vi "Clenshaw.vi"(10 "Cheby weights":dbl[](array[numeric]), 11 "x":dbl) -> (3 "y":dbl)   [LabVIEW 2019]
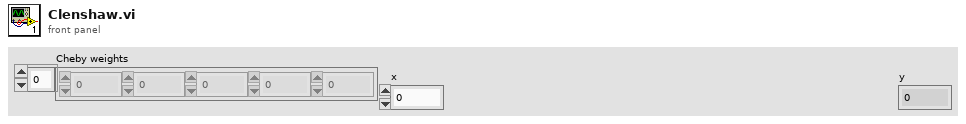
[diagram p1: front panel]
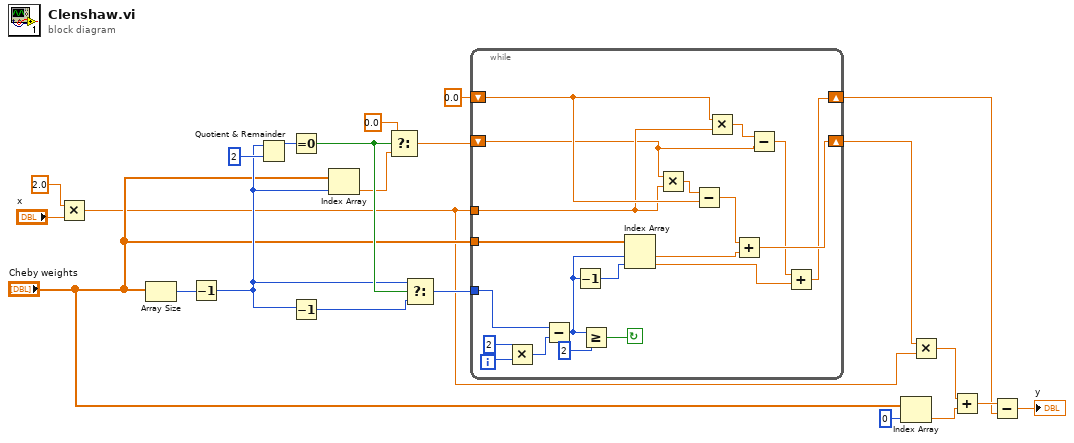
[diagram p0: block diagram]
diagram:
  n1 = Multiply(x=2.0, y="x") -> (x*y=w6:dbl)
  n2 = Array Size(array="Cheby weights") -> (size(s)=w20:i32)
  n3 = Decrement(x=w20) -> (x-1=w11:i32)
  n4 = Quotient & Remainder(x=w11, y=2) -> (x-y*floor(x/y)=w18:i32)  [unwired: 1 out]
  n5 = Equal To 0?(x=w18) -> (x = 0?=w14:bool)
  n6 = Decrement(x=w11) -> (x-1=w13:i32)
  n7 = Index Array(array="Cheby weights", index=w11) -> (element=w10:dbl)
  n8 = Select(t=0.0, s=w14, f=w10) -> (s? t:f=w15:dbl)
  n9 = Select(t=w11, s=w14, f=w13) -> (s? t:f=w12:i32)
  n10 = while {
    tunnel: w6 -> [w27]
    shift-right: [w23] -> w2
    shift-left: 0.0 -> [w28]
    shift-right: [w30] -> w5
    shift-left: w15 -> [w25]
    tunnel: "Cheby weights" -> [w36]
    tunnel: w12 -> [w39]
    i -> [w42]
    stop <- w37 continue-if-true
    n11 = Multiply(x=2, y=w42) -> (x*y=w40:i32)
    n12 = Subtract(x=w39, y=w40) -> (x-y=w34:i32)
    n13 = Decrement(x=w34) -> (x-1=w35:i32)
    n14 = Greater Or Equal?(x=w34, y=2) -> (x >= y?=w37:bool)
    n15 = Index Array(array=w36, index #1=w34, index #2=w35) -> (element #1=w33:dbl, element #2=w29:dbl)
    n16 = Multiply(x=w25, y=w27) -> (x*y=w32:dbl)
    n17 = Subtract(x=w32, y=w28) -> (x-y=w31:dbl)
    n18 = Multiply(x=w28, y=w27) -> (x*y=w26:dbl)
    n19 = Add(x=w31, y=w33) -> (x+y=w30:dbl)
    n20 = Subtract(x=w26, y=w25) -> (x-y=w24:dbl)
    n21 = Add(x=w24, y=w29) -> (x+y=w23:dbl)
  }
  n22 = Index Array(array="Cheby weights", index=0) -> (element=w7:dbl)
  n23 = Multiply(x=w5, y=w6) -> (x*y=w4:dbl)
  n24 = Add(x=w4, y=w7) -> (x+y=w3:dbl)
  n25 = Subtract(x=w3, y=w2) -> (x-y=→"y":dbl)
